vi "Set Output.vi"(8 "error in (no error)":errorcluster, 10 "Output value":refnum<class "Output Value.lvclass">, 11 "Spectrum Recorder in":refnum<class "Spectrum Recorder.lvclass">) -> (0 "error out":errorcluster, 3 "Spectrum Recorder out":refnum<class "Spectrum Recorder.lvclass">)   [LabVIEW 2016, in "Spectrum Recorder.lvclass"]
uses:
  Spectrum Recorder.lvclass
  NHMFL_Core/Libraries/Utilities/Output Value/Output Value.lvclass
  Measure_core/Instrument Actor/Instrument Actor.lvclass
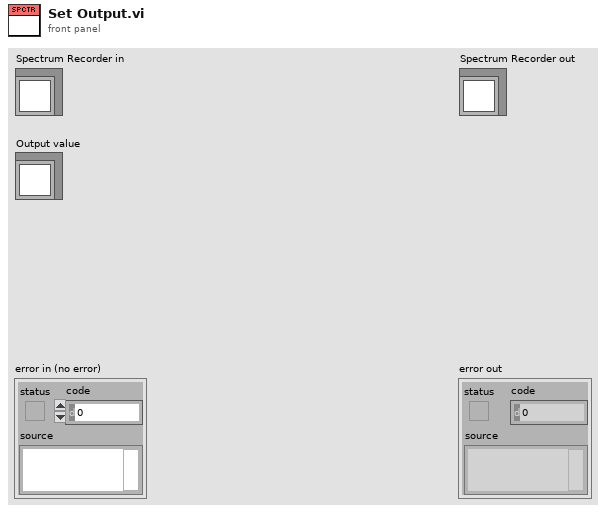
[diagram p1: front panel]
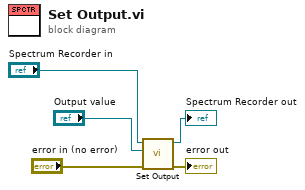
[diagram p0: block diagram]
diagram:
  n1 = call-parent "Set Output.vi"("error in (no error)"="error in (no error)", "Output value"="Output value", "Instrument Actor in"="Spectrum Recorder in") -> ("error out"=→"error out":errorcluster, "Instrument Actor out"=→"Spectrum Recorder out":refnum<class "Spectrum Recorder.lvclass">)  [unwired: 7 in]
